vi "CD Shared lvlib.vi"(8 "error in (no error)":errorcluster, 9 "Action":T1) -> (0 "error out":errorcluster, 1 "Output":string)   [LabVIEW 2014, in "CD model script.lvlib"]
doc: "Constants, which are necessary for the <B>CD Shared library</B> in the generated custom device project."
uses:
  CD model script.lvlib
  Constants TypDef/CD Shared lvlib.ctl
  Constants TypDef/Common.ctl
  Common.vi
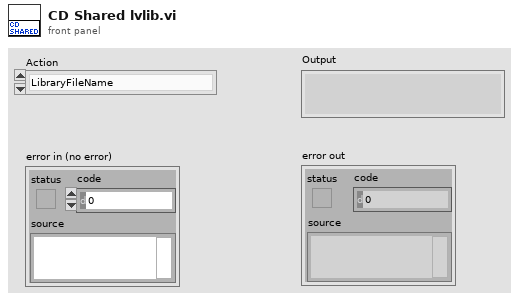
[diagram p1: front panel]
types:
  T1 = typedef "CD model script.lvlib/CD Shared lvlib.ctl" = enum16{"LibraryFileName", "LibraryFolderName", "ConstantsVI.VIPathAndName", "Shared.FolderName", "Shared.Types.FolderName", "Shared.Constants.VIName", "Shared.Constants.VITemplateName", "Shared.Constants.VITemplatePathAndName"}
  T2 = typedef "CD model script.lvlib/Common.ctl" = enum16{"ProjectName", "TemplatesFolderName", "ProjectTemplatePathAndName", "ReadmeTemplatePathAndName", "TimingAndSyncFolderName", "CustomDeviceFolderName"}
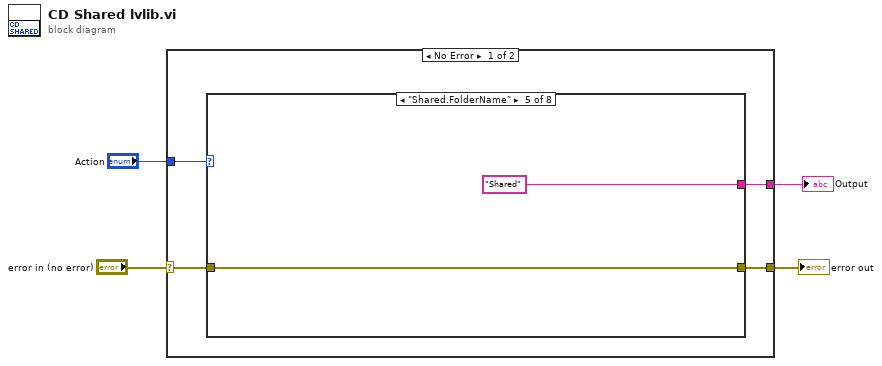
[diagram p0: block diagram]
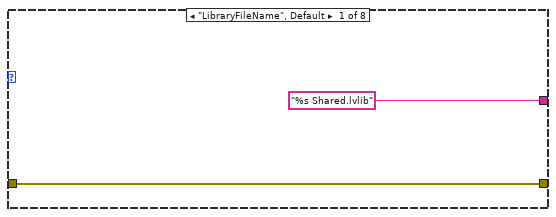
[diagram p2: hidden frame]
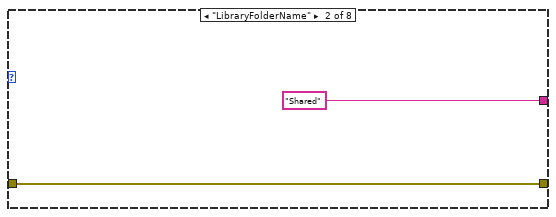
[diagram p3: hidden frame]
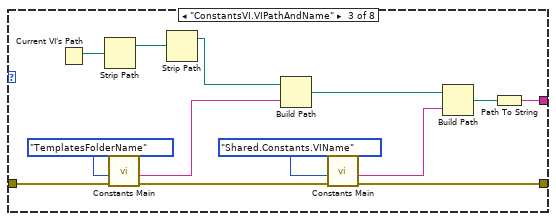
[diagram p4: hidden frame]
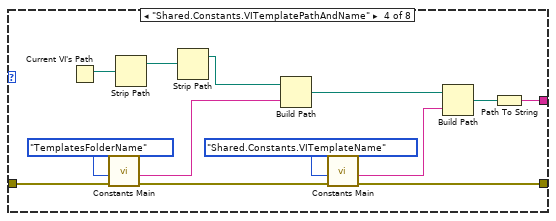
[diagram p5: hidden frame]
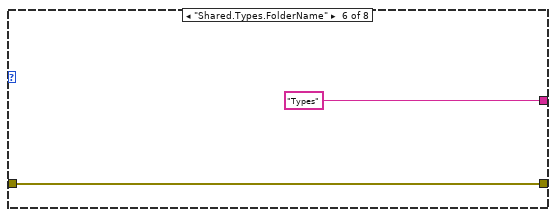
[diagram p6: hidden frame]
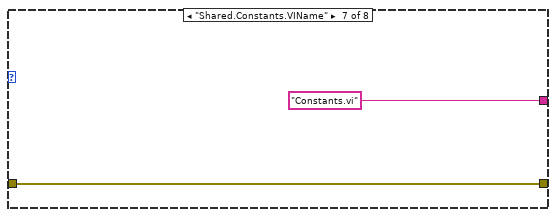
[diagram p7: hidden frame]
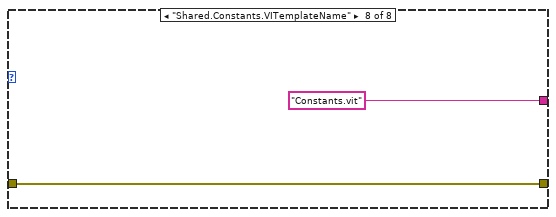
[diagram p8: hidden frame]
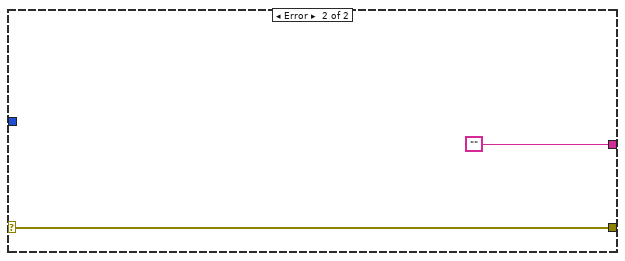
[diagram p9: hidden frame]
diagram:
  n1 = case shown="No Error" "error in (no error)" {
    selector: "error in (no error)" -> [w6 w48]
    tunnel: [w5 w48] -> w3
    tunnel: [w7 ""] -> w2
    tunnel: "Action" -> [w8 _]
    frame No Error {
      n2 = case shown="\"Shared.FolderName\"" w8 {
        tunnel: ["%s Shared.lvlib" "Shared" w25 w38 "Shared" "Types" "Constants.vi" "Constants.vit"] -> w7
        tunnel: w6 -> [w9 w11 w23 w36 w39 w41 w43 w45]
        tunnel: [w9 w11 w17 w30 w39 w41 w43 w45] -> w5
        frame "LibraryFileName", Default {
        }
        frame "LibraryFolderName" {
        }
        frame "ConstantsVI.VIPathAndName" {
          n3 = Current VI's Path() -> (path=w15:path)
          n4 = Strip Path(path=w15) -> (stripped path=w14:path)  [unwired: 1 out]
          n5 = call-poly "Constants Main.vi"("error in (no error)"=w23, "Action"=Common."TemplatesFolderName") -> ("error out"=w18:errorcluster, "Output"=w22:string)  [unwired: 8 in]
          n6 = Strip Path(path=w14) -> (stripped path=w13:path)  [unwired: 1 out]
          n7 = Build Path(base path=w13, name or relative path=w22) -> (appended path=w21:path)
          n8 = call-poly "Constants Main.vi"("error in (no error)"=w18, "Action"=CD_Shared_lvlib."Shared.Constants.VIName") -> ("error out"=w17:errorcluster, "Output"=w16:string)  [unwired: 8 in]
          n9 = Build Path(base path=w21, name or relative path=w16) -> (appended path=w20:path)
          n10 = Path To String(path=w20) -> (string=w25:string)
        }
        frame "Shared.Constants.VITemplatePathAndName" {
          n11 = Current VI's Path() -> (path=w28:path)
          n12 = call-poly "Constants Main.vi"("error in (no error)"=w36, "Action"=Common."TemplatesFolderName") -> ("error out"=w31:errorcluster, "Output"=w35:string)  [unwired: 8 in]
          n13 = Strip Path(path=w28) -> (stripped path=w27:path)  [unwired: 1 out]
          n14 = Strip Path(path=w27) -> (stripped path=w26:path)  [unwired: 1 out]
          n15 = Build Path(base path=w26, name or relative path=w35) -> (appended path=w34:path)
          n16 = call-poly "Constants Main.vi"("error in (no error)"=w31, "Action"=CD_Shared_lvlib."Shared.Constants.VITemplateName") -> ("error out"=w30:errorcluster, "Output"=w29:string)  [unwired: 8 in]
          n17 = Build Path(base path=w34, name or relative path=w29) -> (appended path=w33:path)
          n18 = Path To String(path=w33) -> (string=w38:string)
        }
        frame "Shared.FolderName" {
        }
        frame "Shared.Types.FolderName" {
        }
        frame "Shared.Constants.VIName" {
        }
        frame "Shared.Constants.VITemplateName" {
        }
      }
    }
    frame Error {
    }
  }
  "error out" <- w3
  "Output" <- w2
